vi "Main.vi"(10 "JQMHStartup":refnum<class "RQMHStartup.lvclass">, 11 "TemplateModule in":refnum<class "TemplateModule.lvclass">) -> ()   [LabVIEW 2024, in "TemplateModule.lvclass"]
uses:
  TemplateModule.lvclass
  C:/DevOps/CORTEX/JQMH/JQMHCore/Module/RQMHModule.lvclass
  JQMHCore/JQMHStartup/RQMHStartup.lvclass
  Message Queue_class/RQMHMessageQueue.lvclass/RQMHMessageQueue.ctl
  JQMHCore/Module/InitialiseReplyArgs.ctl
  <vilib>/Utility/miscctls.llb/LVPointTypeDef.ctl
  JQMHCore/Module/RQMHModule.lvclass/RQMHModule.ctl
  Do Something ReplyArgs.ctl
  Do Something Args.ctl
  JamesT ReplyArgs.ctl
  JamesT Args.ctl
  test Args.ctl
  testering Args.ctl
  JQMHCore/Module/RQMHModule.lvclass
  SillySammySau ReplyArgs.ctl
  SillySammySau Args.ctl
  JQMHCore/Module/Read ModuleName.vi
  JQMHCore/Module/Read External Start.vi
  Message Queue_class/Delacor_lib_QMH_Enqueue Message (Single).vi
  Message Queue_class/RQMHMessageQueue.lvclass
  TemplateModule.lvclass/TemplateModule.ctl
  JQMHCore/Shared/RQMHShared.lvlib
panel:
  in  "String":string
  out "error out":errorcluster
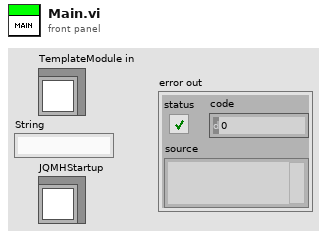
[diagram p1: front panel]
types:
  T1 = typedef "TemplateModule.lvclass/Request Events--cluster.ctl" = cluster{"Do Something":refnum<user-event>, "JamesT":refnum<user-event>, "RRRR":refnum<user-event>, refnum<user-event>, "test":refnum<user-event>, "testering":refnum<user-event>, "SillySammySau":refnum<user-event>}
  T2 = cluster{"Stop Module":refnum<user-event>, "Requests":T1}
  T3 = typedef "LVPointTypeDef.ctl" = cluster{"Horizontal":i16, "Vertical":i16}
  T4 = enum32{"Invalid", "Standard", "Closed", "Hidden", "Minimized", "Maximized"}
  T5 = typedef "RQMHModule.lvclass/InitialiseReplyArgs.ctl" = cluster{"Did Init?":bool}
  T6 = typedef "TemplateModule.lvclass/Do Something Args.ctl" = cluster{"Msg":string}
  T7 = typedef "TemplateModule.lvclass/Do Something ReplyArgs.ctl" = cluster{"Value":dbl, "Boolean":bool}
  T8 = typedef "TemplateModule.lvclass/JamesT Args.ctl" = cluster{"Boolean":bool}
  T9 = typedef "TemplateModule.lvclass/JamesT ReplyArgs.ctl" = cluster{"String":string}
  T10 = typedef "TemplateModule.lvclass/test Args.ctl" = cluster{"String":string}
  T11 = typedef "TemplateModule.lvclass/testering Args.ctl" = cluster{"RQMHModule.lvclass":refnum<class "RQMHModule.lvclass">}
  T12 = typedef "TemplateModule.lvclass/SillySammySau Args.ctl" = cluster{"Boolean":bool}
  T13 = typedef "TemplateModule.lvclass/SillySammySau ReplyArgs.ctl" = cluster{"String":string}
  T14 = typedef "RQMHModule.lvclass/Reply.ctl" = cluster{"Expects Reply":bool, "Reply":refnum<notifier>}
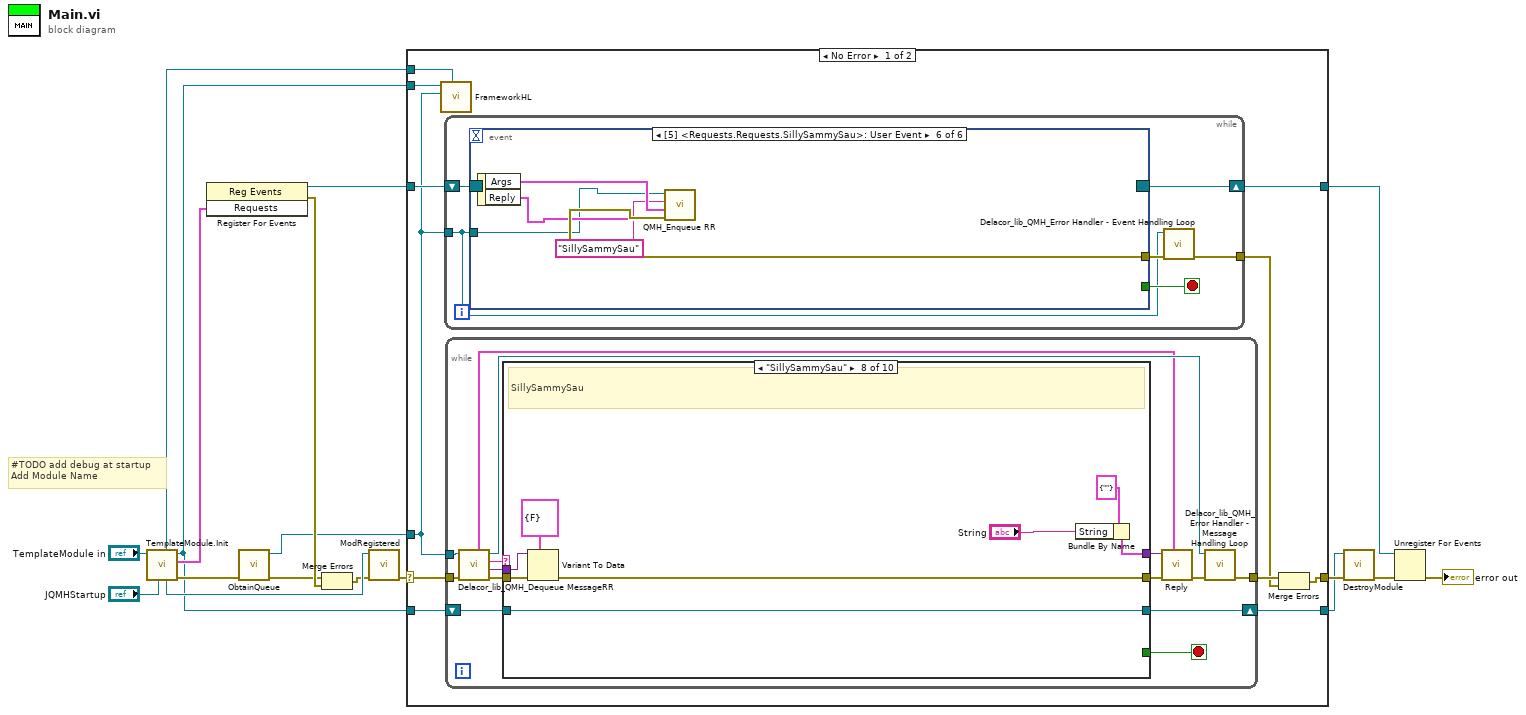
[diagram p0: block diagram]
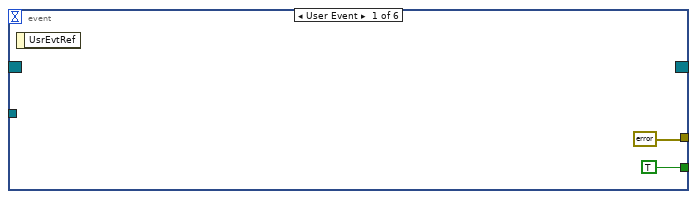
[diagram p2: hidden frame]
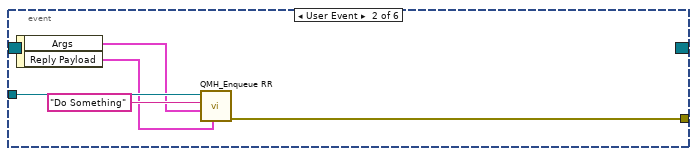
[diagram p3: hidden frame]
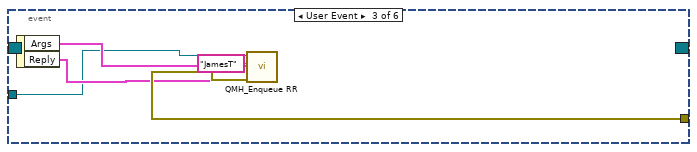
[diagram p4: hidden frame]
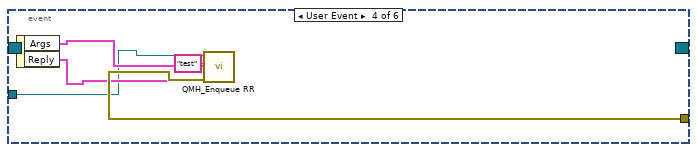
[diagram p5: hidden frame]
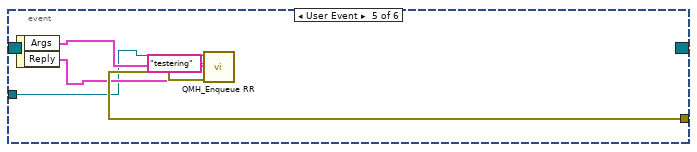
[diagram p6: hidden frame]
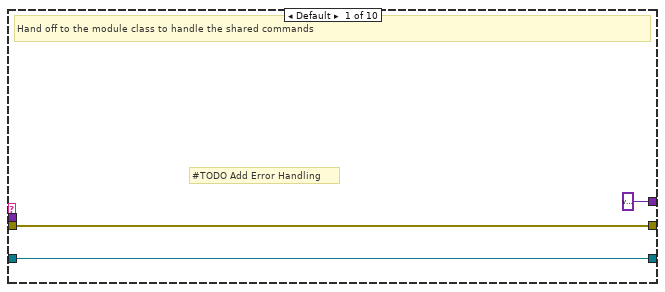
[diagram p7: hidden frame]
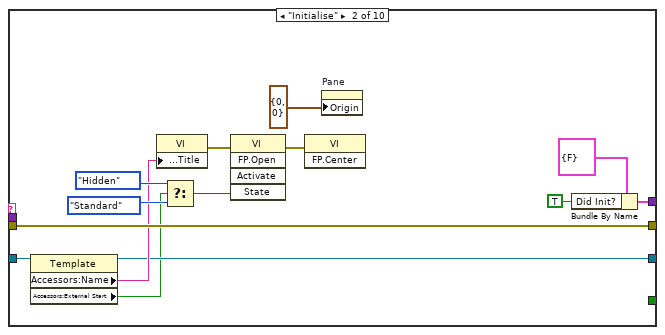
[diagram p8: hidden frame]
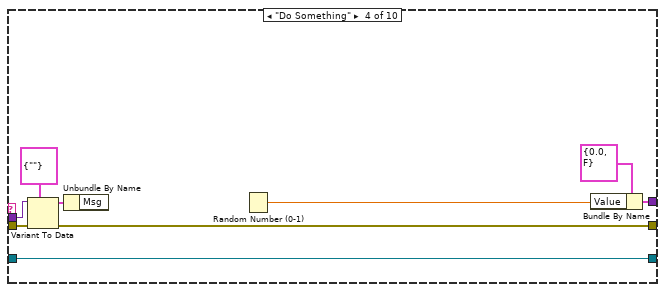
[diagram p10: hidden frame]
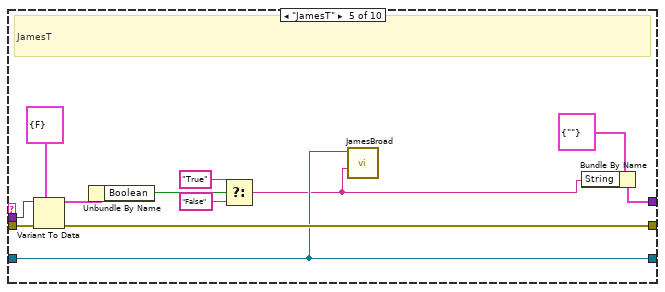
[diagram p11: hidden frame]
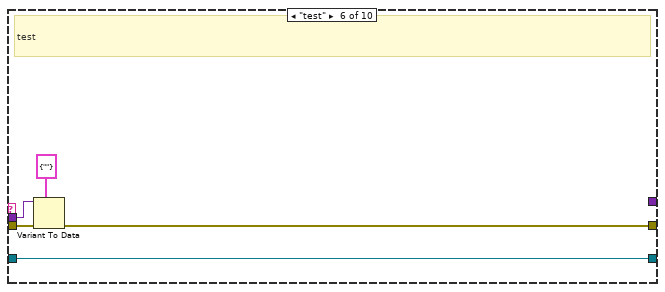
[diagram p12: hidden frame]
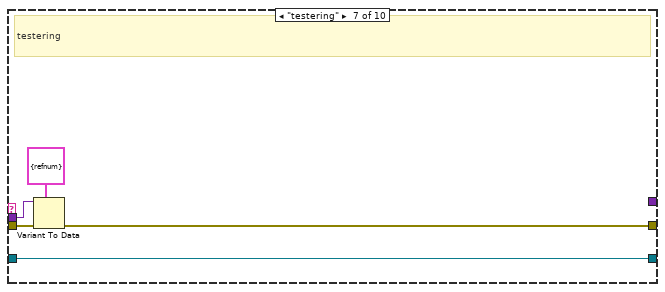
[diagram p13: hidden frame]
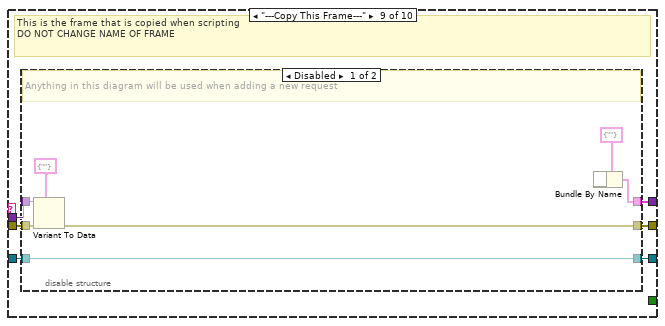
[diagram p14: hidden frame]
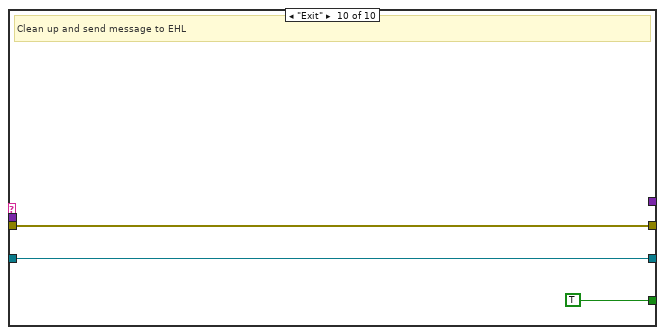
[diagram p16: hidden frame]
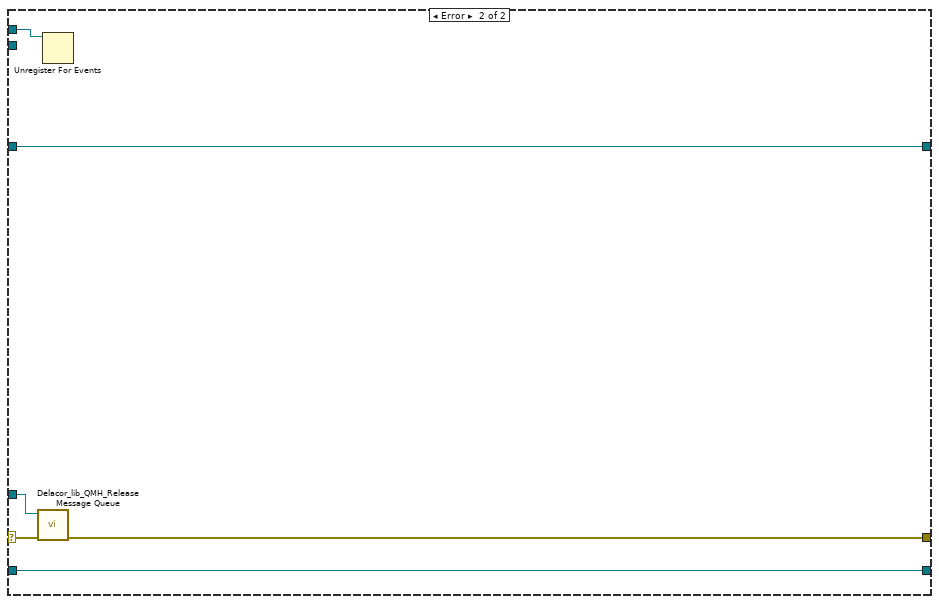
[diagram p17: hidden frame]
diagram:
  # "#TODO add debug at startup\nAdd Module Name"
  n1 = call "TemplateModule.Init.vi"("JQMHStartup in"="JQMHStartup", "TemplateModule in"="TemplateModule in") -> ("error out"=w11:errorcluster, "Requests"=w2:T2, "TemplateModule out"=w1:refnum<class "TemplateModule.lvclass">, "JQMHStartup out"=w9:refnum<class "RQMHStartup.lvclass">, "StandardRequests"=w5:refnum<event-registration>)  [unwired: 4 in, 1 out]
  n2 = register-events(w2) -> (reference out=w4:refnum<event-registration>, error out=w18:errorcluster)  [unwired: 2 in]
  n3 = call "ObtainQueue.vi"("error in"=w11) -> ("error out"=w10:errorcluster, "Message Queue"=w6:refnum<class "RQMHMessageQueue.lvclass">)  [unwired: 9 in]
  n4 = Merge Errors(w10, w18) -> (w7:errorcluster)
  n5 = call "ModRegistered.vi"("error in (no error)"=w7, "JQMHStartup in"=w9) -> ("error out"=w8:errorcluster)  [unwired: 9 in]
  n6 = case "RQMH_MAIN" shown="No Error" w8 {
    selector: w8 -> [w26 w156]
    tunnel: w1 -> [w29 w155]
    tunnel: [w28 w158] -> w17
    tunnel: w4 -> [w27 w158]
    tunnel: w6 -> [w20 w157]
    tunnel: [w25 w155] -> w3
    tunnel: [w22 w154] -> w14
    tunnel: w1 -> [w21 _]
    tunnel: w5 -> [w19 w153]
    frame No Error {
      n7 = call-dynamic "FrameworkHL.vi"("StandardRequests"=w19, "Message Queue"=w20, "JQMHModule in"=w21) -> ()  [unwired: 9 in]
      n8 = while {
        shift-right: [w35] -> w28
        shift-left: w27 -> [w30]
        tunnel: w20 -> [w31]
        tunnel: [w32] -> w23
        stop <- w34 stop-if-true
        n9 = event "RQMH_EVENT_MAIN" shown="[5] <Requests.Requests.SillySammySau>: User Event" {
          selector: w30 -> [_ _ _ _ _ _]
          dyn-events: [_ _ _ _ _ _] -> w35
          timeout: _ -> [_ _ _ _ _ _]
          tunnel: [TRUE _ _ _ _ _] -> w34
          tunnel: w31 -> [_ w42 w44 w49 w54 w59]
          tunnel: [errorcluster {"status"=FALSE, "code"=0, "source"=""} ("error out") w39 w47 w52 w57 w62] -> w33
          event User Event {
            n10 = event-data() -> ()  [unwired: 1 in, 1 out]
          }
          event User Event {
            n11 = event-data() -> ("Args"=w40:T6, "Reply Payload"=w38:T14)  [unwired: 1 in]
            n12 = call "QMH_Enqueue RR.vi"("Reply"=w38, "Message Data"=w40, "Message"="Do Something", "Message Queue in"=w42) -> ("error out"=w39:errorcluster)  [unwired: 6 in, 1 out]
          }
          event User Event {
            n13 = event-data() -> ("Args"=w45:T8, "Reply"=w46:T14)  [unwired: 1 in]
            n14 = call "QMH_Enqueue RR.vi"("Reply"=w46, "Message Data"=w45, "Message"="JamesT", "Message Queue in"=w44) -> ("error out"=w47:errorcluster)  [unwired: 6 in, 1 out]
          }
          event User Event {
            n15 = event-data() -> ("Args"=w50:T10, "Reply"=w51:T14)  [unwired: 1 in]
            n16 = call "QMH_Enqueue RR.vi"("Reply"=w51, "Message Data"=w50, "Message"="test", "Message Queue in"=w49) -> ("error out"=w52:errorcluster)  [unwired: 6 in, 1 out]
          }
          event User Event {
            n17 = event-data() -> ("Args"=w55:T11, "Reply"=w56:T14)  [unwired: 1 in]
            n18 = call "QMH_Enqueue RR.vi"("Reply"=w56, "Message Data"=w55, "Message"="testering", "Message Queue in"=w54) -> ("error out"=w57:errorcluster)  [unwired: 6 in, 1 out]
          }
          event User Event {
            n19 = event-data() -> ("Args"=w60:T12, "Reply"=w61:T14)  [unwired: 1 in]
            n20 = call "QMH_Enqueue RR.vi"("Reply"=w61, "Message Data"=w60, "Message"="SillySammySau", "Message Queue in"=w59) -> ("error out"=w62:errorcluster)  [unwired: 6 in, 1 out]
          }
        }
        n21 = call-dynamic "Delacor_lib_QMH_Error Handler - Event Handling Loop.vi"("error in"=w33, "Message Queue in"=w31) -> ("dup error in"=w32:errorcluster)  [unwired: 8 in, 1 out]
      }
      n22 = while {
        tunnel: w20 -> [w71]
        tunnel: w26 -> [w70]
        shift-right: [w73] -> w25
        shift-left: w29 -> [w74]
        tunnel: [w72] -> w24
        stop <- w76 stop-if-true
        n23 = call-dynamic "Delacor_lib_QMH_Dequeue MessageRR.vi"("error in"=w70, "Message Queue in"=w71) -> ("error out"=w69:errorcluster, "Message Data"=w67:variant, "Message"=w68:string, "Message Queue out"=w75:refnum<class "RQMHMessageQueue.lvclass">, "Reply"=w63:T14)  [unwired: 5 in]
        n24 = case "RQMH_MESSAGE_CASES" shown="\"SillySammySau\"" w68 {
          tunnel: [_ _ _ _ _ _ _ _ _ TRUE] -> w76
          tunnel: w74 -> [w78 w81 w94 w104 w112 w119 w124 w132 w138 w151]
          tunnel: w67 -> [_ _ _ w100 w114 w118 w123 w131 w136 _]
          tunnel: w69 -> [w79 w93 w95 w99 w116 w121 w126 w134 w140 w150]
          tunnel: [w79 w93 w95 w98 w115 w120 w125 w133 w139 w150] -> w66
          tunnel: [w78 w82 w94 w104 w112 w119 w124 w132 w137 w151] -> w73
          tunnel: [variant w92 _ w103 w113 _ _ w130 w135 _] -> w64
          frame Default {
            # "#TODO Add Error Handling"
            # "Hand off to the module class to handle the shared commands"
          }
          frame "Initialise" {
            n25 = property class="Template"(reference=w81) -> (reference out=w82:refnum<class "TemplateModule.lvclass">, "Accessors:Name"=w83:string, "Accessors:External Start"=w80:bool)  [unwired: 1 in, 1 out]
            n26 = property on="Property Node" class="VI"("Front Panel.Title"=w83) -> (error out=w90:errorcluster)  [unwired: 2 in, 1 out]
            n27 = Select(t=T4."Hidden" ("State"), s=w80, f=T4."Standard" ("State")) -> (s? t:f=w86:T4)
            n28 = invoke on="Invoke Node" class="VI" method="FP.Open"(error in=w90, "State"=w86) -> (error out=w89:errorcluster)  [unwired: 3 in, 4 out]
            n29 = invoke on="Invoke Node" class="VI" method="FP.Center"(error in=w89) -> ()  [unwired: 2 in, 3 out]
            n30 = property on="Pane" class="Pane"("Origin"=T3 {"Horizontal"=0, "Vertical"=0}) -> ()  [unwired: 2 in, 2 out]
            n31 = Bundle By Name(cluster=T5 {"Did Init?"=FALSE} ("Args"), "Did Init?"=TRUE) -> (w92:T5)
          }
          frame "---Module Specific---" {
          }
          frame "Do Something" {
            n32 = Variant To Data(error in=w99, type=T6 {"Msg"=""} ("Do Something Args"), Variant=w100) -> (data=w96:T6, error out=w98:errorcluster)
            n33 = Unbundle By Name(w96) -> ()  [unwired: 1 out]
            n34 = Random Number (0-1)() -> (number: 0 to 1=w101:dbl)
            n35 = Bundle By Name(cluster=T7 {"Value"=0.0, "Boolean"=FALSE}, "Value"=w101) -> (w103:T7)
          }
          frame "JamesT" {
            # "JamesT"
            n36 = Variant To Data(error in=w116, type=T8 {"Boolean"=FALSE} ("Args"), Variant=w114) -> (data=w111:T8, error out=w115:errorcluster)
            n37 = Unbundle By Name(w111) -> ("Boolean"=w110:bool)
            n38 = Select(t="True", s=w110, f="False") -> (s? t:f=w106:string)
            n39 = call "JamesBroad.vi"("String"=w106, "TemplateModule in"=w112) -> ()  [unwired: 8 in, 2 out]
            n40 = Bundle By Name(cluster=T9 {"String"=""} ("RQMH_MHL_REPLY_PL"), "String"=w106) -> (w113:T9)
          }
          frame "test" {
            # "test"
            n41 = Variant To Data(error in=w121, type=T10 {"String"=""} ("RQMH_MHL_MSG_PL"), Variant=w118) -> (error out=w120:errorcluster)  [unwired: 1 out]
          }
          frame "testering" {
            # "testering"
            n42 = Variant To Data(error in=w126, type=T11 {"RQMHModule.lvclass"=refnum} ("RQMH_MHL_MSG_PL"), Variant=w123) -> (error out=w125:errorcluster)  [unwired: 1 out]
          }
          frame "SillySammySau" {
            # "SillySammySau"
            n43 = Variant To Data(error in=w134, type=T12 {"Boolean"=FALSE} ("RQMH_MHL_MSG_PL"), Variant=w131) -> (error out=w133:errorcluster)  [unwired: 1 out]
            n44 = Bundle By Name(cluster=T13 {"String"=""} ("RQMH_MHL_REPLY_PL"), "String"="String") -> (w130:T13)
          }
          frame "---Copy This Frame---" {
            # "This is the frame that is copied when scripting\nDO NOT CHANGE NAME OF FRAME"
            n45 = disable-structure shown="Disabled" {
              disable-tunnel: w140 -> [w144 w149]
              disable-tunnel: [w145 w149] -> w139
              disable-tunnel: w138 -> [w147 w148]
              disable-tunnel: [w147 w148] -> w137
              disable-tunnel: w136 -> [w146 _]
              disable-tunnel: [w142 _] -> w135
              frame Disabled {
                # "Anything in this diagram will be used when adding a new request"
                n46 = Variant To Data(error in=w144, type=cluster{string} {""} ("RQMH_MHL_MSG_PL"), Variant=w146) -> (error out=w145:errorcluster)  [unwired: 1 out]
                n47 = Bundle By Name(cluster=cluster{string} {""} ("RQMH_MHL_REPLY_PL")) -> (w142:cluster{string})  [unwired: 1 in]
              }
              frame Enabled {
              }
            }
          }
          frame "Exit" {
            # "Clean up and send message to EHL"
          }
        }
        n48 = call "Reply.vi"("Reply"=w63, "error in (no error)"=w66, "ReplyPayload"=w64) -> ("error out"=w65:errorcluster)  [unwired: 8 in]
        n49 = call-dynamic "Delacor_lib_QMH_Error Handler - Message Handling Loop.vi"("error in"=w65, "Message Queue in"=w75) -> ("dup error in"=w72:errorcluster)  [unwired: 8 in, 1 out]
      }
      n50 = Merge Errors(w24, w23) -> (w22:errorcluster)
    }
    frame Error {
      n51 = call-dynamic "Delacor_lib_QMH_Release Message Queue.vi"("error in"=w156, "Message Queue"=w157) -> ("error out"=w154:errorcluster)  [unwired: 9 in]
      n52 = Unregister For Events(event registration refnum=w153) -> ()  [unwired: 1 in, 1 out]
    }
  }
  n53 = call "DestroyModule.vi"("error in (no error)"=w14, "JQMHModule in"=w3) -> ("error out"=w16:errorcluster)  [unwired: 9 in]
  n54 = Unregister For Events(event registration refnum=w17, error in=w16) -> (error out=→"error out":errorcluster)
